vi "Inpterpolate4_complement.vi"(0 "X":fxp<+/-,16,14>, 11 "input valid":bool=TRUE) -> (4 "X(t)":fxp<+/-,16,14>, 6 "X(t -1)":fxp<+/-,16,14>, 8 "X(t -2)":fxp<+/-,16,14>, 10 "X(t -3)":fxp<+/-,16,14>, 15 "output valid":bool)   [LabVIEW 2018]
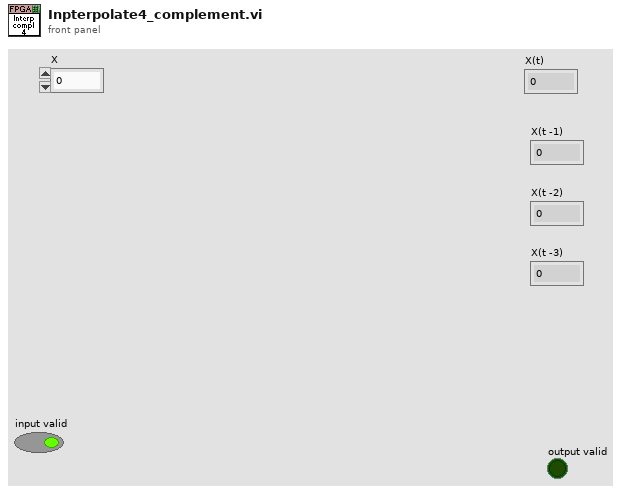
[diagram p1: front panel]
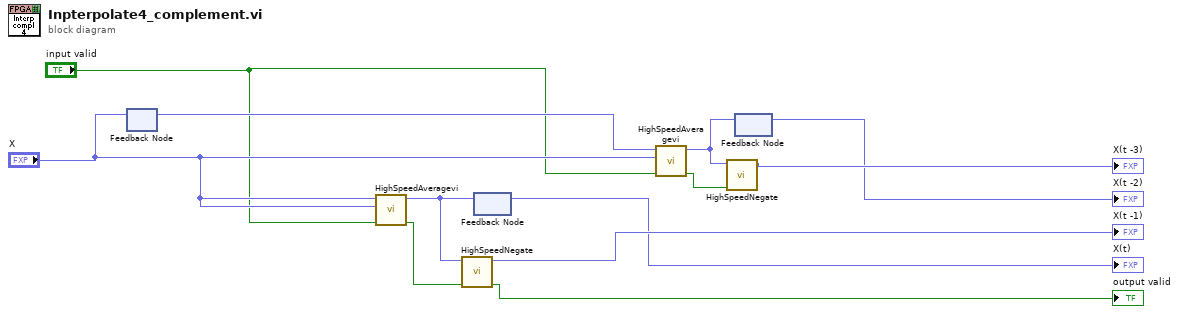
[diagram p0: block diagram]
diagram:
  n1 = feedback #1() -> (w12:fxp<+/-,16,14>)  [unwired: 1 in]
  n2 = feedback-in #1("X") -> ()
  n3 = call "HighSpeedAveragevi.vi"("input valid"="input valid", "y"="X", "x"="X") -> ("output valid"=w10:bool, "(x+y)/2"=w8:fxp<+/-,16,14>)  [unwired: 7 in]
  n4 = call "HighSpeedNegate.vi"("input valid"=w10, "x"=w8) -> ("output valid"=→"output valid":bool, "-x"=→"X(t -1)":fxp<+/-,16,14>)  [unwired: 8 in]
  n5 = feedback #2() -> (→"X(t)":fxp<+/-,16,14>)  [unwired: 1 in]
  n6 = feedback-in #2(w8) -> ()
  n7 = call "HighSpeedAveragevi.vi"("input valid"="input valid", "y"="X", "x"=w12) -> ("output valid"=w11:bool, "(x+y)/2"=w4:fxp<+/-,16,14>)  [unwired: 7 in]
  n8 = call "HighSpeedNegate.vi"("input valid"=w11, "x"=w4) -> ("-x"=→"X(t -3)":fxp<+/-,16,14>)  [unwired: 8 in, 1 out]
  n9 = feedback #3() -> (→"X(t -2)":fxp<+/-,16,14>)  [unwired: 1 in]
  n10 = feedback-in #3(w4) -> ()
